vi "CardChannel2MuxChannel.vi"(0 "Probecard Channel No.":i32=1 min=1 max=32 step=1) -> (1 "Mux No. string":string, 2 "Mux No.:":u32(ring)=1 items=["", "", "", "", "MUX1", "MUX2"], 3 "C1 / C2":i32=1 min=1 max=2 step=1, 4 "Channel":i32=1 min=1 max=8 step=1)   [LabVIEW 2013]
uses:
  general_VIs/globals/QC_MeasurementSetup.vi
  InstrControl/InstrumentSetup.vi
  InstrControl/InstrControl.lvclass
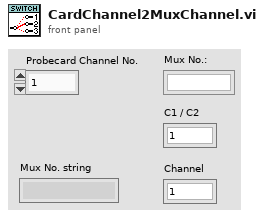
[diagram p1: front panel]
types:
  T1 = cluster{"Bias Supply":refnum<class "SupplyControl.lvclass">, "SMU":refnum<class "SupplyControl.lvclass">, "LCR":refnum<class "LCRControl.lvclass">, "Probe Card Channels":i32, "Bias Voltage [V]":dbl, "First strip":i32, "Last strip":i32, "Base Voltage [V]":dbl, "Base Ramp Step [V]":dbl, "Base Ramp Interval [ms]":u32, "High Voltage [V]":dbl, "High Ramp Step [V]":dbl, "High Ramp Interval [ms]":u32, "Single Needle":bool, "ArduinoControl.lvclass":refnum<class "ArduinoControl.lvclass">, "Fraction of good strips [%]":dbl}
  T2 = cluster{"GPIB address":string, "Matrix address":string, "Mux1 address":string, "Mux2 address":string, "Matrix used?":bool, "Switching":refnum<class "Switching.lvclass">, "Matrix X Channels":cluster{"Bias Supply / SMU LO":i32, "Bias Supply / SMU HI":i32, "CV Box LO":i32, "CV Box HI":i32, "CV Box LO IN":i32, "CV Box HI IN":i32, "Volt meter LO":i32, "Volt meter HI":i32, "Mux1 C1":i32, "Mux1 C2":i32, "Mux2 C1":i32, "Mux2 C2":i32}}
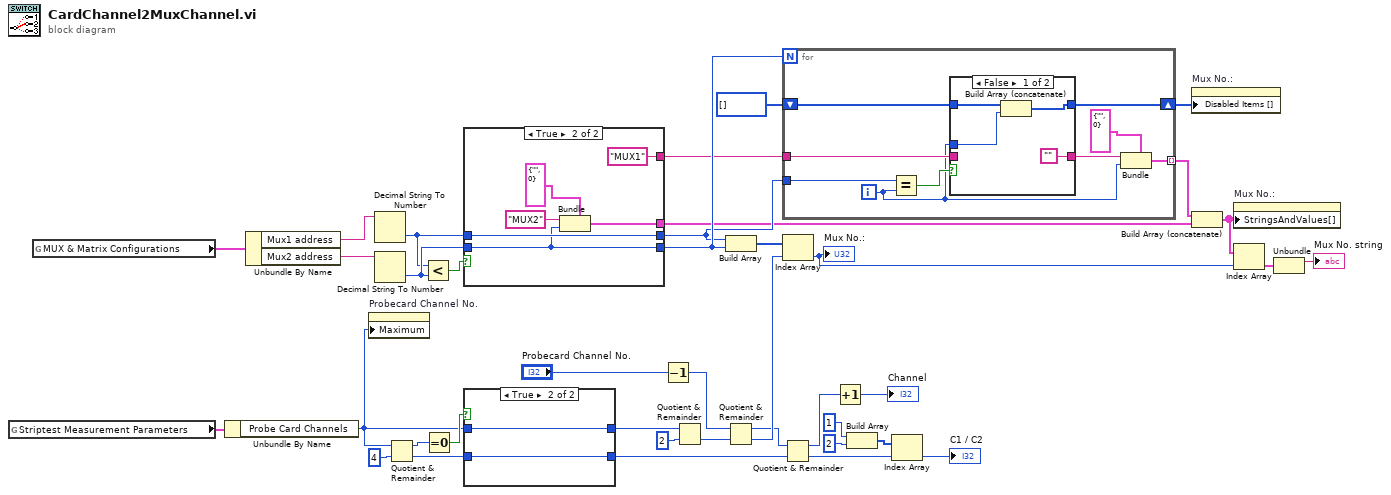
[diagram p0: block diagram]
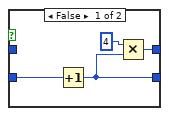
[diagram p2: hidden frame]
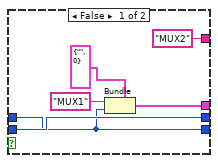
[diagram p3: hidden frame]
diagram:
  n1 = global read "QC_MeasurementSetup.vi" "Striptest Measurement Parameters"() -> (w9:T1)
  n2 = global read "InstrumentSetup.vi" "MUX & Matrix Configurations"() -> (w7:T2)
  n3 = Unbundle By Name(w9) -> ("Probe Card Channels"=w8:i32)
  n4 = Unbundle By Name(w7) -> ("Mux1 address"=w6:string, "Mux2 address"=w5:string)
  n5 = property on="Probecard Channel No." class="DigNum (strict)"("Maximum"=w8) -> ()  [unwired: 2 in, 2 out]
  n6 = Decimal String To Number(string=w6) -> (number=w11:i32)  [unwired: 2 in, 1 out]
  n7 = Decimal String To Number(string=w5) -> (number=w12:i32)  [unwired: 2 in, 1 out]
  n8 = Quotient & Remainder(x=w8, y=4) -> (x-y*floor(x/y)=w27:i32, floor(x/y)=w29:i32)
  n9 = Less?(x=w11, y=w12) -> (x < y?=w10:bool)
  n10 = Equal To 0?(x=w27) -> (x = 0?=w26:bool)
  n11 = case shown="True" w10 {
    tunnel: w11 -> [w42 w51]
    tunnel: w12 -> [w44 w47]
    tunnel: [w44 w51] -> w31
    tunnel: [w42 w47] -> w32
    tunnel: ["MUX2" "MUX1"] -> w13
    tunnel: [w41 w46] -> w17
    frame False {
      n12 = Bundle(cluster=cluster{string, i32} {"", 0}, "MUX1", w42) -> (w41:cluster{string, i32})
    }
    frame True {
      n13 = Bundle(cluster=cluster{string, i32} {"", 0}, "MUX2", w47) -> (w46:cluster{string, i32})
    }
  }
  n14 = case shown="True" w26 {
    tunnel: w8 -> [_ w57]
    tunnel: [w55 w57] -> w28
    tunnel: w29 -> [w54 w56]
    tunnel: [w52 w56] -> w30
    frame False {
      n15 = Increment(x=w54) -> (x+1=w52:i32)
      n16 = Multiply(x=4, y=w52) -> (x*y=w55:i32)
    }
    frame True {
    }
  }
  n17 = Decrement(x="Probecard Channel No.") -> (x-1=w21:i32)
  n18 = Quotient & Remainder(x=w28, y=2) -> (floor(x/y)=w22:i32)  [unwired: 1 out]
  n19 = Build Array(w31, w32) -> (w33:i32[])
  n20 = Quotient & Remainder(x=w21, y=w22) -> (x-y*floor(x/y)=w25:i32, floor(x/y)=w34:i32)
  n21 = for {
    N: w32 -> [_]
    tunnel: [w65] -> w16 mode=indexing
    tunnel: w31 -> [w63]
    tunnel: w13 -> [w62]
    shift-right: [w60] -> w14
    shift-left: i32[] [] -> [w58]
    i -> [w59]
    n22 = Equal?(x=w63, y=w59) -> (x = y?=w66:bool)
    n23 = case shown="False" w66 {
      tunnel: w62 -> [_ w72]
      tunnel: ["" w72] -> w61
      tunnel: [w68 w71] -> w60
      tunnel: w59 -> [w69 _]
      tunnel: w58 -> [w67 w71]
      frame False {
        n24 = Build Array (concatenate)(w67, w69) -> (w68:i32[])
      }
      frame True {
      }
    }
    n25 = Bundle(cluster=cluster{string, i32} {"", 0}, w61, w59) -> (w65:cluster{string, i32})
  }
  n26 = Index Array(array=w33, index=w34) -> (element=w3:i32)
  "Mux No.:" <- w3
  n27 = Quotient & Remainder(x=w25, y=w30) -> (x-y*floor(x/y)=w24:i32, floor(x/y)=w38:i32)
  n28 = Increment(x=w24) -> (x+1=→"Channel":i32)
  n29 = Build Array(1, 2) -> (w37:i32[])
  n30 = Index Array(array=w37, index=w38) -> (element=→"C1 / C2":i32)
  n31 = property on="Mux No.:" class="Ring (strict)"("Disabled Items []"=w14) -> ()  [unwired: 2 in, 2 out]
  n32 = Build Array (concatenate)(w16, w17) -> (w4:cluster{string, i32}[])
  n33 = property on="Mux No.:" class="Ring (strict)"("StringsAndValues[]"=w4) -> ()  [unwired: 2 in, 2 out]
  n34 = Index Array(array=w4, index=w3) -> (element=w2:cluster{string, i32})
  n35 = Unbundle(w2) -> (→"Mux No. string":string)  [unwired: 1 out]
